vi "Write Sub Panel Products.vi"(8 "error in (no error)":errorcluster, 10 "Sub Panel Products":refnum<vi>, 11 "Coca Actor in":refnum<class "Coca Actor.lvclass">) -> (0 "error out":errorcluster, 3 "Coca Actor out":refnum<class "Coca Actor.lvclass">)   [LabVIEW 2020, in "Coca Actor.lvlib" / "Coca Actor.lvclass"]
uses:
  Coca Actor.lvclass
  Coca Actor.lvclass/Coca Actor.ctl
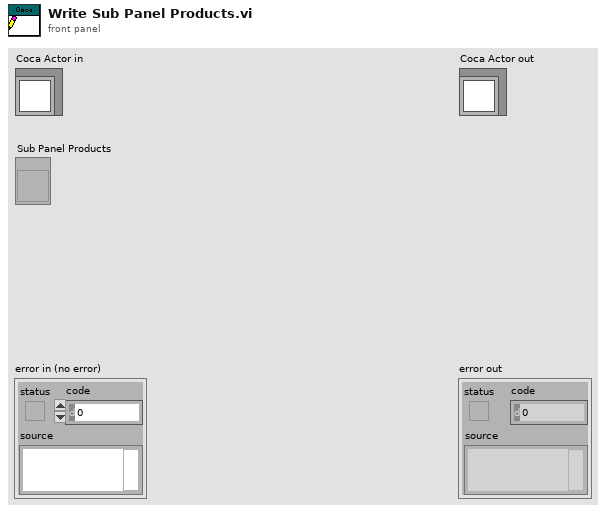
[diagram p1: front panel]
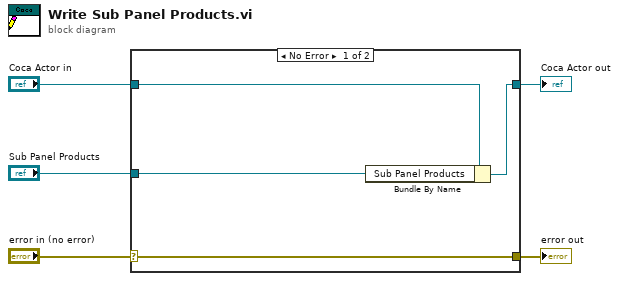
[diagram p0: block diagram]
diagram:
  n1 = case shown="No Error" "error in (no error)" {
    selector: "error in (no error)" -> [w9 w10]
    tunnel: [w9 w10] -> w4
    tunnel: [w7 w11] -> w2
    tunnel: "Coca Actor in" -> [w8 w11]
    tunnel: "Sub Panel Products" -> [w6 _]
    frame No Error {
      n2 = Bundle By Name(cluster=w8, "Sub Panel Products"=w6) -> (w7:refnum<class "Coca Actor.lvclass">)
    }
    frame Error {
    }
  }
  "error out" <- w4
  "Coca Actor out" <- w2
